vi "save_udc_config_file.vi"(1 "Config File":path, 2 "Value Array":dbl[](array[numeric]), 3 "UDC Table":string[][](array[string])) -> ()   [LabVIEW 2011]
panel:
  out "Error Out":errorcluster caption="error out"
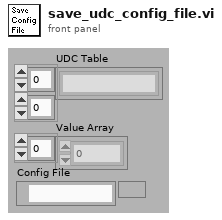
[diagram p1: front panel]
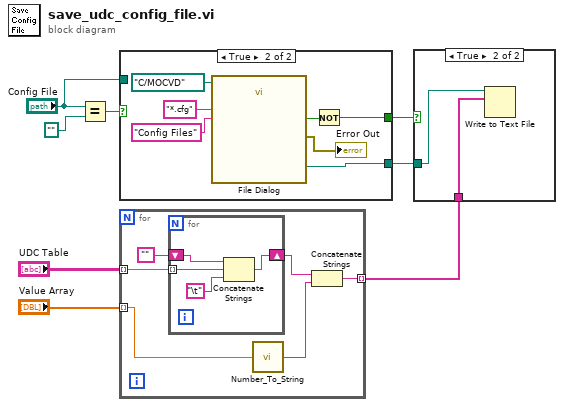
[diagram p0: block diagram]
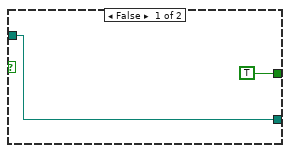
[diagram p3: hidden frame]
diagram:
  n1 = Equal?(x="Config File", y=path "") -> (x = y?=w5:bool)
  n2 = case shown="True" w5 {
    tunnel: [TRUE w12] -> w4
    tunnel: [w10 w13] -> w3
    tunnel: "Config File" -> [w10 _]
    frame False {
    }
    frame True {
      n3 = call "File Dialog"("start path"=path "C:/MOCVD", "pattern (all files)"="*.cfg", "pattern label"="Config Files") -> ("selected path"=w13:path, "cancelled"=w14:bool, "error out"=→"Error Out":errorcluster)  [unwired: 4 in, 6 out]
      n4 = Not(x=w14) -> (.not. x?=w12:bool)
    }
  }
  n5 = for {
    tunnel: "UDC Table" -> [w23] mode=indexing
    tunnel: "Value Array" -> [w20] mode=indexing
    tunnel: [w19] -> w1 mode=indexing
    n6 = for {
      tunnel: w23 -> [w27] mode=indexing
      shift-right: [w25] -> w21
      shift-left: "" -> [w26]
      n7 = Concatenate Strings(w26, w27, "\t") -> (w25:string)
    }
    n8 = call "Number_To_String.vi"("Number"=w20) -> ("String"=w18:string)
    n9 = Concatenate Strings(w21, w18) -> (w19:string)
  }
  n10 = case shown="True" w4 {
    tunnel: w3 -> [_ w29]
    tunnel: w1 -> [_ w28]
    frame False {
    }
    frame True {
      n11 = Write to Text File(file (use dialog)=w29, text=w28) -> ()  [unwired: 1 in, 4 out]
    }
  }
